vi "ReadDVRTracepoint.vi"(6 "found":bool, 7 "Qbus":refnum<class "Qbus.lvclass">, 8 "DVR":u32, 9 "element location":u32, 10 "Requested Location":u32, 11 "source":string) -> ()   [LabVIEW 2017]
uses:
  <vilib>/addons/Qbus/Qbus.lvclass
  <vilib>/addons/TraceLogger/TraceLogger.lvlib
  <vilib>/addons/InsightCM/Devices/Shared/Common/DataAccumulator/DataAccumulator.lvlib
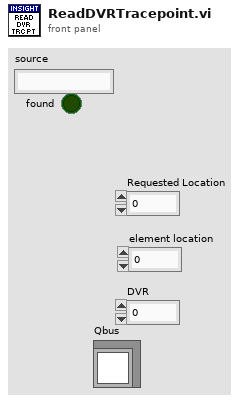
[diagram p1: front panel]
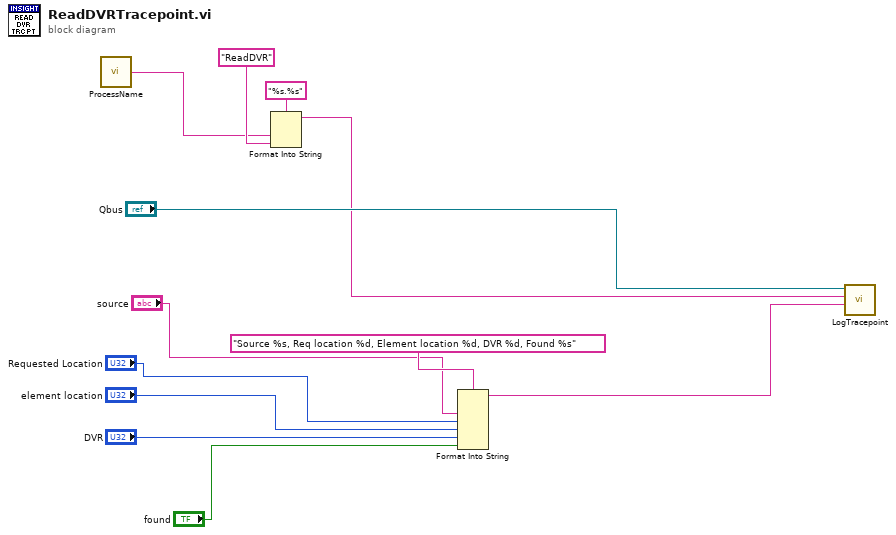
[diagram p0: block diagram]
diagram:
  n1 = call <vilib>:"ProcessName.vi"() -> ("process name"=w1:string)  [unwired: 5 in]
  n2 = Format Into String(format string="%s.%s", w1, "ReadDVR" ("tracepoint")) -> (resulting string=w8:string)  [unwired: 2 in, 1 out]
  n3 = Format Into String(format string="Source %s, Req location %d, Element location %d, DVR %d, Found %s", "source", "Requested Location", "element location", "DVR", "found") -> (resulting string=w5:string)  [unwired: 2 in, 1 out]
  n4 = call <vilib>:"LogTracepoint.vi"("log string"=w5, "tracepoint"=w8, "qbus in"="Qbus") -> ()  [unwired: 7 in, 2 out]
